vi "Read Board.vi"(11 "Position in":refnum<class "Position.lvclass">) -> (2 "Chesslib.lvlib:Board.lvclass":refnum<class "Board.lvclass">, 3 "Position out":refnum<class "Position.lvclass">)   [LabVIEW 2015, in "Chesslib.lvlib" / "Position.lvclass"]
uses:
  Position.lvclass
  Board/Board.lvclass
  Position.lvclass/Position.ctl
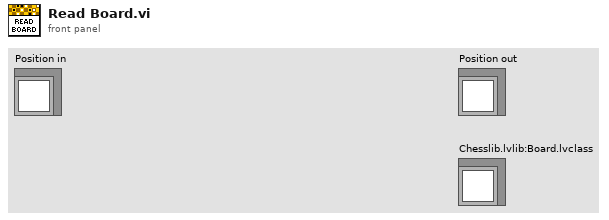
[diagram p1: front panel]
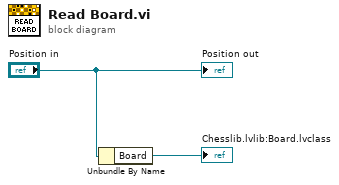
[diagram p0: block diagram]
diagram:
  n1 = Unbundle By Name("Position in") -> ("Board"=→"Chesslib.lvlib:Board.lvclass":refnum<class "Board.lvclass">)
  "Position out" <- "Position in"
